vi "Read Delimiters.vi"(8 "Error In":errorcluster, 11 "Token In":refnum<class "Token.lvclass">) -> (0 "Error Out":errorcluster, 2 "Delimiters":T1, 3 "Token Out":refnum<class "Token.lvclass">)   [LabVIEW 2018, in "Toolkit.lvlib" / "Tokens.lvlib" / "Token.lvclass"]
doc: "Gets the opening and closing components that surround, or delimit, a Mustache tag."
uses:
  Token.lvclass
  Type Definitions/Delimiters.ctl
  Token.lvclass/Token.ctl
  Toolkit.lvlib
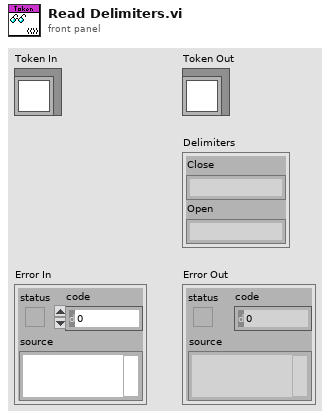
[diagram p1: front panel]
types:
  T1 = typedef "Toolkit.lvlib/Delimiters.ctl" = cluster{"Close":string, "Open":string}
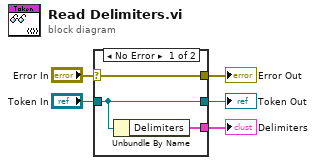
[diagram p0: block diagram]
diagram:
  n1 = case shown="No Error" "Error In" {
    selector: "Error In" -> [w8 w10]
    tunnel: [w8 w10] -> w4
    tunnel: [w7 w9] -> w2
    tunnel: "Token In" -> [w7 w9]
    tunnel: [w6 _] -> w1
    frame No Error {
      n2 = Unbundle By Name(w7) -> ("Delimiters"=w6:T1)
    }
    frame Error {
    }
  }
  "Error Out" <- w4
  "Token Out" <- w2
  "Delimiters" <- w1
